vi "Pre Launch Init.vi"(11 "Nested in":refnum<class "UserConsole.lvclass">) -> (0 "error out":errorcluster, 3 "Nested out":refnum<class "UserConsole.lvclass">)   [LabVIEW 2025, in "UserConsole.lvlib" / "UserConsole.lvclass"]
doc: "(<B>Filename</B>: Actor Framework.lvlib:Actor.lvclass:Pre Launch Init.vi)\n\nDefines behavior that occurs after the Launch Nested Actor method is invoked but before the actor's Actor Core method begins running.\n\nBy default, this method does nothing. A descendant class may override it to define behavior."
uses:
  UserConsole.lvclass
  C:/Program Files (x86)/National Instruments/LabVIEW 2025/vi.lib/ActorFramework/Actor/Actor.lvclass
  UserConsole.lvclass/UserConsole.ctl
  <vilib>/ActorFramework/Actor/Actor.lvclass/Actor.ctl
  UserConsole Messages/Case-Controller Msg/Case-Controller Msg.lvclass/Case-Controller Msg.ctl
  <vilib>/ActorFramework/Message Enqueuer/Message Enqueuer.lvclass/Message Enqueuer.ctl
  <vilib>/ActorFramework/Message Enqueuer/Enqueue.vi
  UserConsole Messages/Case-Controller Msg/Case-Controller Msg.lvclass
  C:/Program Files (x86)/National Instruments/LabVIEW 2025/vi.lib/ActorFramework/Message/Message.lvclass
  <vilib>/ActorFramework/Message Priority Queue/Priority Enqueue.vi
  <vilib>/ActorFramework/Actor/Actor.lvclass
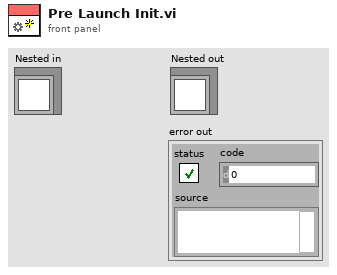
[diagram p1: front panel]
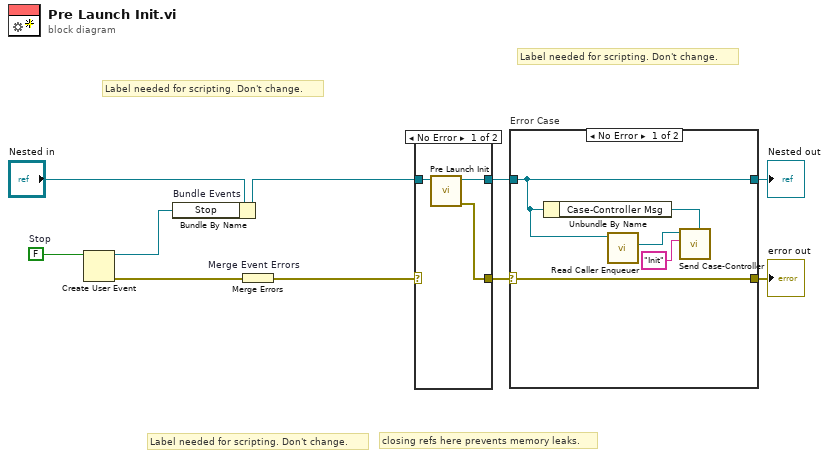
[diagram p0: block diagram]
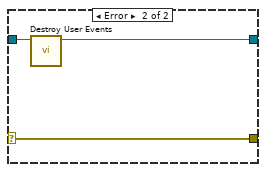
[diagram p3: hidden frame]
diagram:
  w9 = FALSE  # Stop
  # "Label needed for scripting. Don't change."
  # "Label needed for scripting. Don't change."
  # "Label needed for scripting. Don't change."
  # "closing refs here prevents memory leaks."
  n1 = Create User Event(user event datatype=w9) -> (user event=w7:refnum<user-event>, error out=w8:errorcluster)  [unwired: 1 in]
  n2 = Bundle By Name "Bundle Events"(cluster="Nested in", "Stop"=w7) -> (w4:refnum<class "UserConsole.lvclass">)
  n3 = Merge Errors "Merge Event Errors"(w8) -> (w3:errorcluster)
  n4 = case shown="No Error" w3 {
    selector: w3 -> [_ w15]
    tunnel: [w13 w14] -> w5
    tunnel: w4 -> [w12 w14]
    tunnel: [w11 w15] -> w2
    frame No Error {
      n5 = call-parent "Pre Launch Init.vi"("Actor in"=w12) -> ("error out"=w11:errorcluster, "Actor out"=w13:refnum<class "UserConsole.lvclass">)  [unwired: 9 in]
    }
    frame Error {
    }
  }
  n6 = case "Error Case" shown="No Error" w2 {
    selector: w2 -> [w20 w23]
    tunnel: w5 -> [w18 w22]
    tunnel: [w18 w21] -> w1
    tunnel: [w20 w23] -> w6
    frame No Error {
      n7 = Unbundle By Name(w18) -> ("Case-Controller Msg"=w19:refnum<class "Case-Controller Msg.lvclass">)
      n8 = call <vilib>:"Read Caller Enqueuer.vi"("Actor"=w18) -> ("Caller Enqueuer"=w17:refnum<class "Message Enqueuer.lvclass">)  [unwired: 10 in]
      n9 = call "Send Case-Controller.vi"("Message Type"=w19, "Controller Case"="Init", "Message Enqueuer"=w17) -> ()  [unwired: 7 in, 2 out]
    }
    frame Error {
      n10 = call "Destroy User Events.vi"("UI Template in"=w22) -> ("UI Template out"=w21:refnum<class "UserConsole.lvclass">)  [unwired: 10 in]
    }
  }
  "error out" <- w6
  "Nested out" <- w1
